vi "LaserState.vi"(8 "Laser state":bool, 10 "Laser":refnum<vi>, 11 "Laser side":T1) -> ()   [LabVIEW 2018]
uses:
  laserSide.ctl
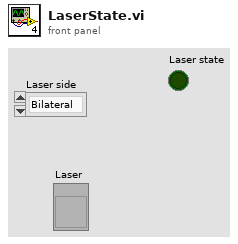
[diagram p1: front panel]
types:
  T1 = typedef "laserSide.ctl" = enum16{"Bilateral", "Left", "Right"}
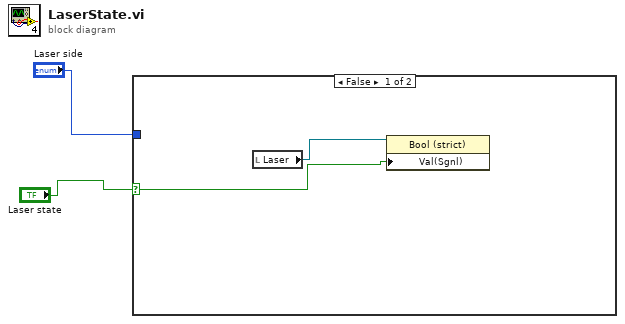
[diagram p0: block diagram]
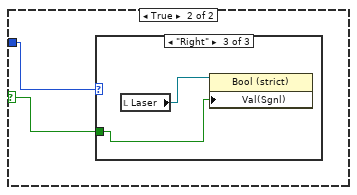
[diagram p2: hidden frame]
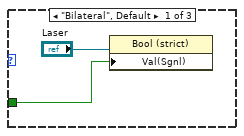
[diagram p3: hidden frame]
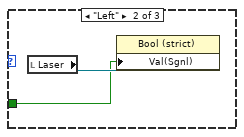
[diagram p4: hidden frame]
diagram:
  n1 = case shown="False" "Laser state" {
    selector: "Laser state" -> [w3 w6]
    tunnel: "Laser side" -> [_ w5]
    frame False {
      n2 = local read "Laser"() -> (w4:refnum<vi>)
      n3 = property class="Bool (strict)"(reference=w4, "Val(Sgnl)"=w3) -> ()  [unwired: 1 in, 2 out]
    }
    frame True {
      n4 = case shown="\"Right\"" w5 {
        tunnel: w6 -> [w7 w9 w12]
        frame "Bilateral", Default {
          n5 = property class="Bool (strict)"(reference="Laser", "Val(Sgnl)"=w7) -> ()  [unwired: 1 in, 2 out]
        }
        frame "Left" {
          n6 = local read "Laser"() -> (w10:refnum<vi>)
          n7 = property class="Bool (strict)"(reference=w10, "Val(Sgnl)"=w9) -> ()  [unwired: 1 in, 2 out]
        }
        frame "Right" {
          n8 = local read "Laser"() -> (w11:refnum<vi>)
          n9 = property class="Bool (strict)"(reference=w11, "Val(Sgnl)"=w12) -> ()  [unwired: 1 in, 2 out]
        }
      }
    }
  }
